vi "string-hexstring-313.vi"(11 "字符串":string) -> (3 "十六进制整型字符串":string)   [LabVIEW 2016]
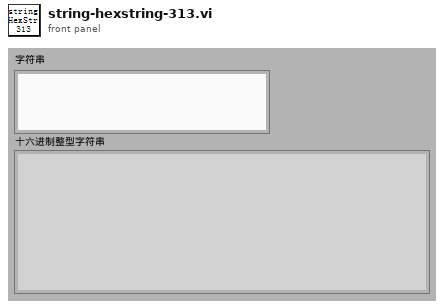
[diagram p1: front panel]
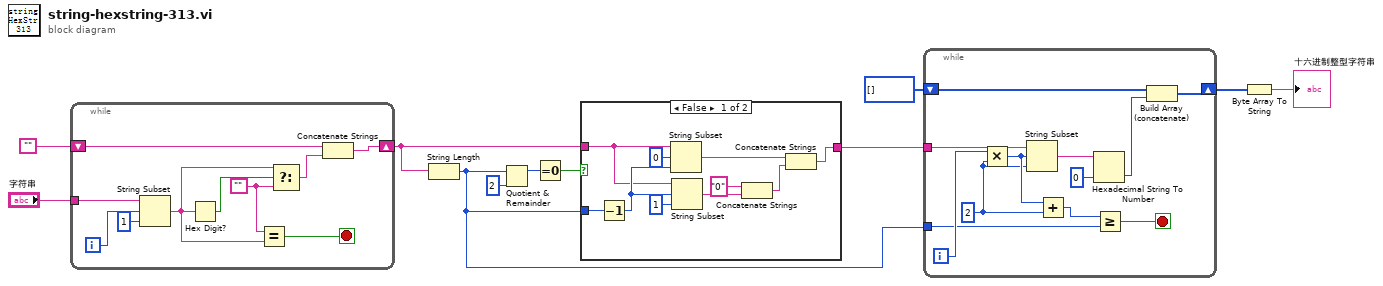
[diagram p0: block diagram]
diagram:
  n1 = while {
    tunnel: "字符串" -> [w20]
    shift-right: [w14] -> w6
    shift-left: "" -> [w16]
    i -> [w19]
    stop <- w18 stop-if-true
    w12 = ""
    n2 = String Subset(string=w20, offset (0)=w19, length (rest)=1 ("length (rest)")) -> (substring=w15:string)
    n3 = Hex Digit?(1:w15) -> (0:w17:bool)
    n4 = Equal?(x=w12, y=w15) -> (x = y?=w18:bool)
    n5 = Select(t=w15, s=w17, f=w12) -> (s? t:f=w13:string)
    n6 = Concatenate Strings(w16, w13) -> (w14:string)
  }
  n7 = String Length(string=w6) -> (length=w1:i32)
  n8 = Quotient & Remainder(x=w1, y=2) -> (x-y*floor(x/y)=w8:i32)  [unwired: 1 out]
  n9 = Equal To 0?(x=w8) -> (x = 0?=w7:bool)
  n10 = case shown="False" w7 {
    tunnel: w6 -> [w24 w32]
    tunnel: w1 -> [w23 _]
    tunnel: [w22 w32] -> w5
    frame False {
      n11 = Decrement(x=w23) -> (x-1=w26:i32)
      n12 = String Subset(string=w24, offset (0)=0, length (rest)=w26) -> (substring=w30:string)
      n13 = String Subset(string=w24, offset (0)=w26, length (rest)=1 ("length (rest)")) -> (substring=w28:string)
      n14 = Concatenate Strings("0", w28) -> (w31:string)
      n15 = Concatenate Strings(w30, w31) -> (w22:string)
    }
    frame True {
    }
  }
  n16 = while {
    shift-right: [w39] -> w3
    shift-left: u8[] [] -> [w38]
    tunnel: w5 -> [w44]
    tunnel: w1 -> [w36]
    i -> [w43]
    stop <- w33 stop-if-true
    w35 = 2
    n17 = Multiply(x=w43, y=w35) -> (x*y=w37:i32)
    n18 = String Subset(string=w44, offset (0)=w37, length (rest)=w35) -> (substring=w41:string)
    n19 = Add(x=w37, y=w35) -> (x+y=w34:i32)
    n20 = Hexadecimal String To Number(string=w41, default (0uL)=u8 0) -> (number=w40:u8)  [unwired: 1 in, 1 out]
    n21 = Greater Or Equal?(x=w34, y=w36) -> (x >= y?=w33:bool)
    n22 = Build Array (concatenate)(w38, w40) -> (w39:u8[])
  }
  n23 = Byte Array To String(unsigned byte array=w3) -> (string=→"十六进制整型字符串":string)
